vi "Relative ns to Double Seconds.vi"(4 "relative ns":i64) -> (7 "Double s":dbl)   [LabVIEW 2020, in "Vecto.lvlib"]
uses:
  Vecto.lvlib
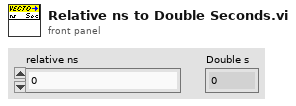
[diagram p1: front panel]
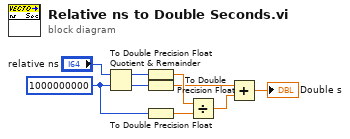
[diagram p0: block diagram]
diagram:
  w6 = i64 1000000000 ("y")
  n1 = Quotient & Remainder(x="relative ns", y=w6) -> (x-y*floor(x/y)=w7:i64, floor(x/y)=w8:i64)
  n2 = To Double Precision Float(number=w7) -> (double precision float=w4:dbl)
  n3 = To Double Precision Float(number=w8) -> (double precision float=w3:dbl)
  n4 = To Double Precision Float(number=w6) -> (double precision float=w5:dbl)
  n5 = Divide(x=w4, y=w5) -> (x/y=w2:dbl)
  n6 = Add(x=w3, y=w2) -> (x+y=→"Double s":dbl)
